vi "Pre Post File Path.vi"(4 "Extension":string, 6 "Post":string, 9 "Pre":string, 10 "Rename Library File Path":path) -> (1 "Post File Path":path, 2 "Pre File Path":path)   [LabVIEW 2020, in "_Rename.lvlib" / "_Rename.lvclass"]
uses:
  _Rename.lvclass
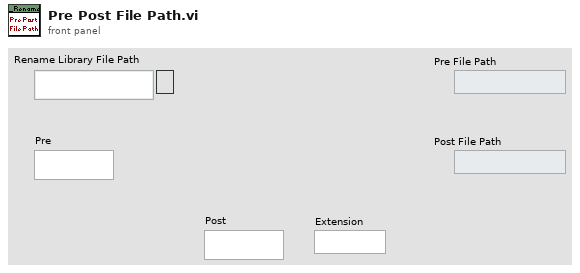
[diagram p1: front panel]
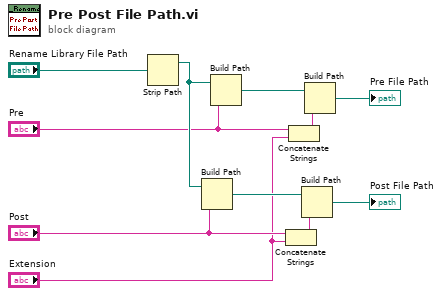
[diagram p0: block diagram]
diagram:
  n1 = Strip Path(path="Rename Library File Path") -> (stripped path=w6:path)  [unwired: 1 out]
  n2 = Build Path(base path=w6, name or relative path="Post") -> (appended path=w10:path)
  n3 = Build Path(base path=w6, name or relative path="Pre") -> (appended path=w8:path)
  n4 = Concatenate Strings("Post", "Extension") -> (w11:string)
  n5 = Concatenate Strings("Pre", "Extension") -> (w9:string)
  n6 = Build Path(base path=w10, name or relative path=w11) -> (appended path=→"Post File Path":path)
  n7 = Build Path(base path=w8, name or relative path=w9) -> (appended path=→"Pre File Path":path)
